vi "SQL_UpdateToolCribPrice.vi"   [LabVIEW 2017]
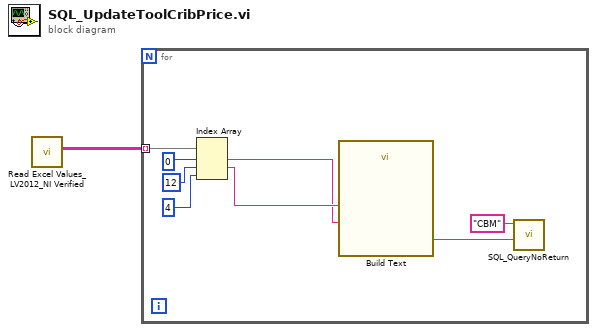
[diagram p0: block diagram]
diagram:
  n1 = call "Read Excel Values_LV2012_NI Verified.vi"() -> ("ExcelData"=w1:string[][])  [unwired: 11 in]
  n2 = for {
    tunnel: w1 -> [w9] mode=indexing
    n3 = Index Array(array=w9, index #1=0, index #2=12, index #3=4) -> (element #1=w2:string, element #2=w3:string)  [unwired: 1 out]
    n4 = call "Build Text"("price"=w3, "toolcribpn"=w2) -> ("Result"=w6:string)  [unwired: 12 in, 1 out]
    n5 = call "SQL_QueryNoReturn.vi"("SQL query"=w6, "ConnectionDSN"="CBM") -> ()  [unwired: 10 in]
  }
